vi "set io cond list.vi"(8 "error in (no error)":errorcluster, 9 "mask_set":u16, 10 "mask_0":u16, 11 "mask_1":u16) -> (0 "error out":errorcluster)   [LabVIEW 2015, in "SCANalone4x64.lvlib"]
doc: "__declspec(dllimport) void __stdcall set_io_cond_list(unsigned short mask_1, unsigned short mask_0, unsigned short mask_set);"
uses:
  <userlib>/SCANalone4x64/SCANalone4x64.lvlib
  <userlib>/SCANalone4x64/SCANalone4x64.dll
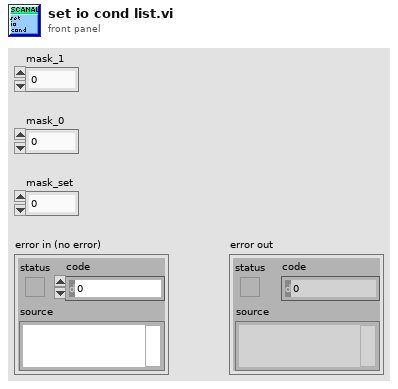
[diagram p1: front panel]
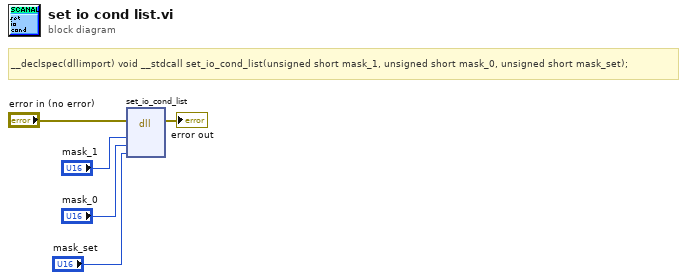
[diagram p0: block diagram]
diagram:
  # "__declspec(dllimport) void __stdcall set_io_cond_list(unsigned short mask_1, unsigned short mask_0, unsigned short mask_set);"
  n1 = dll-call lib="C:/Program Files/National Instruments/LabVIEW 2015/user.lib/SCANalone4x64/SCANalone4x64.*" fn="set_io_cond_list"(error in="error in (no error)", "mask_1"="mask_1", "mask_0"="mask_0", "mask_set"="mask_set") -> (error out=→"error out":errorcluster)  [unwired: 6 in, 1 out]
